vi "BNC555.evt call Chan Mode.vi"(0 "i ref in":refnum<vi>, 2 "Generator Instance":string="N/A", 3 "Channel":i32(ring)=1 items=["System (To)", "Channel A", "Channel B", "Channel C", "Channel D", "Channel E", "Channel F", "Channel G", "Channel H"], 4 "Mode":T1(ring), 5 "error in (no error)":errorcluster, 7 "Burst # (10)":u32=10, 9 "Divide # (10)":u32=10) -> (14 "i ref out":refnum<vi>, 19 "error out":errorcluster)   [LabVIEW 2014, in "BNC555.lvlib"]
doc: "This VI sends a simple event call to the wired BNC555."
uses:
  BNC555.lvlib
  CS_Core/CSSystem/CoreLib/CoreLib.int 2 byte array.vi
  CS_Core/CSSystem/CoreLib/CoreLib.short 2 byte array.vi
  CS_Core/CSSystem/CoreLib/CoreLib.lvlib
  CS_Core/BaseProcess/BaseProcess.lvlib
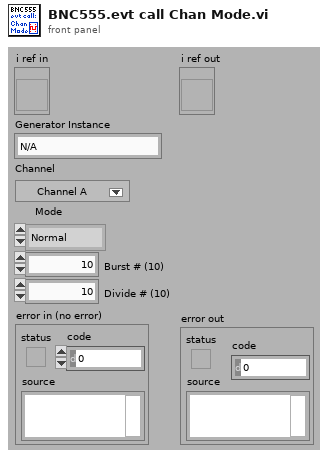
[diagram p1: front panel]
types:
  T1 = enum16{"Normal", "Single", "Burst", "Divide by N"}
  T2 = typedef "CoreDefs.rawDataType.ctl" = i8[]
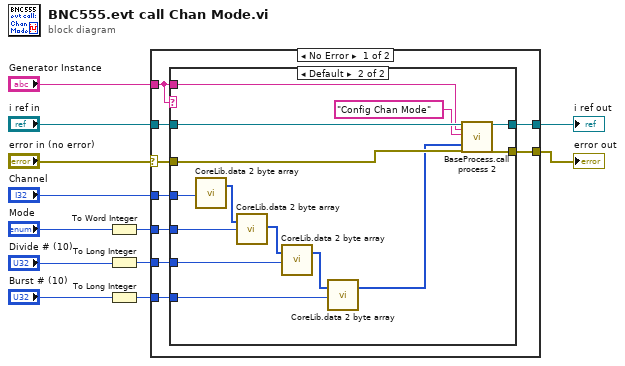
[diagram p0: block diagram]
diagram:
  n1 = To Word Integer(number="Mode") -> (16bit integer=w6:i16)
  n2 = To Long Integer(number="Divide # (10)") -> (32bit integer=w5:i32)
  n3 = To Long Integer(number="Burst # (10)") -> (32bit integer=w1:i32)
  n4 = case shown="No Error" "error in (no error)" {
    selector: "error in (no error)" -> [w18 w38]
    tunnel: [w21 w39] -> w11
    tunnel: [w20 w38] -> w10
    tunnel: "i ref in" -> [w19 w39]
    tunnel: "Generator Instance" -> [w17 _]
    tunnel: "Channel" -> [w16 _]
    tunnel: w6 -> [w15 _]
    tunnel: w5 -> [w14 _]
    tunnel: w1 -> [w13 _]
    frame No Error {
      n5 = case shown="Default" w17 {
        tunnel: [w23 w37] -> w21
        tunnel: [w22 w36] -> w20
        tunnel: w19 -> [w23 w35]
        tunnel: w17 -> [_ w34]
        tunnel: w18 -> [w22 w32]
        tunnel: w16 -> [_ w31]
        tunnel: w15 -> [_ w30]
        tunnel: w14 -> [_ w25]
        tunnel: w13 -> [_ w24]
        frame "N/A" {
        }
        frame Default {
          n6 = call-poly "CoreLib.data 2 byte array.vi"("i32"=w31) -> ("byteArray out"=w29:T2)  [unwired: 18 in]
          n7 = call-poly "CoreLib.data 2 byte array.vi"("byteArray"=w29, "i16"=w30) -> ("byteArray out"=w27:T2)  [unwired: 17 in]
          n8 = call-poly "CoreLib.data 2 byte array.vi"("byteArray"=w27, "i32"=w25) -> ("byteArray out"=w28:T2)  [unwired: 17 in]
          n9 = call-poly "CoreLib.data 2 byte array.vi"("byteArray"=w28, "i32"=w24) -> ("byteArray out"=w26:T2)  [unwired: 17 in]
          n10 = call "BaseProcess.call process 2.vi"("i ref in"=w35, "Object"=w34, "Selector"="Config Chan Mode", "Data"=w26, "error in (no error)"=w32) -> ("i ref out"=w37:refnum<vi>, "error out"=w36:errorcluster)  [unwired: 13 in]
        }
      }
    }
    frame Error {
    }
  }
  "error out" <- w10
  "i ref out" <- w11
